vi "Start Polling.vi"(8 "error in (no error)":errorcluster, 11 "Zero Timeout Message Handler in":refnum<class "Zero Timeout Message Handler.lvclass">) -> (0 "error out":errorcluster, 3 "Zero Timeout Message Handler out":refnum<class "Zero Timeout Message Handler.lvclass">)   [LabVIEW 2024, in "Zero Timeout Message Handler.lvlib" / "Zero Timeout Message Handler.lvclass"]
uses:
  Zero Timeout Message Handler.lvclass
  Zero Timeout Message Handler.lvclass/Zero Timeout Message Handler.ctl
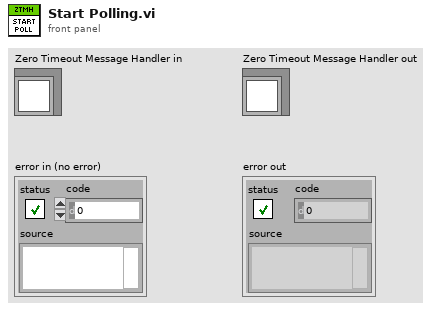
[diagram p1: front panel]
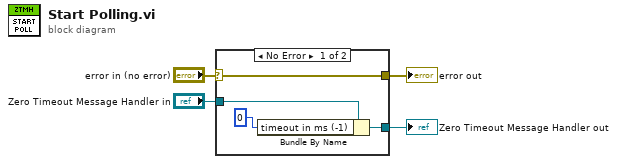
[diagram p0: block diagram]
diagram:
  n1 = case shown="No Error" "error in (no error)" {
    selector: "error in (no error)" -> [w8 w10]
    tunnel: [w8 w10] -> w3
    tunnel: [w6 w9] -> w1
    tunnel: "Zero Timeout Message Handler in" -> [w7 w9]
    frame No Error {
      n2 = Bundle By Name(cluster=w7, "timeout in ms (-1)"=0) -> (w6:refnum<class "Zero Timeout Message Handler.lvclass">)
    }
    frame Error {
    }
  }
  "error out" <- w3
  "Zero Timeout Message Handler out" <- w1
